vi "RT Driver VI.vi"(6 "Device Clock":string, 9 "Device Inputs FIFO":refnum<k33>, 10 "Device Outputs FIFO":refnum<k33>, 11 "Device Reference":T1 format="%.0x") -> ()   [LabVIEW 2016, in "UDP Sender Engine.lvlib"]
uses:
  UDP Sender Engine.lvlib
  <vilib>/NI Veristand/Custom Device API/Custom Device Item Ref.ctl
  <vilib>/NI Veristand/Custom Device API/Custom Device Channel Type.ctl
  Shared/Constants.vi
  <vilib>/NI Veristand/Custom Device API/Get Item Property (String).vi
  <vilib>/NI Veristand/Custom Device API/Get Item Property (U16).vi
  <vilib>/NI Veristand/Custom Device API/Custom Device API.lvlib
  <vilib>/NI Veristand/Custom Device Tools/Custom Device Utility Library/Custom Device Utility Library.lvlib
  Shared/UDP Sender Shared.lvlib
panel:
  in  "Initialization Status Notifier":refnum<notifier>
  in  "Status Notifier":refnum<notifier>
  # "Custom Device Template\nv1.0"
  # "Use this template as a starting point for creating a custom device code module. The input controls shown here are specially named controls that the system will use to provide the device loop with data. The controls are not required for the device loop to run. For instance, if the device doesn't produce any output data, then you don't need the Device Outputs FIFO control. If you do use these controls, however, they need to have these exact names to be functional."
  # "The optional status notifier element is used to notify the RT engine of the last state of the custom device, and to indicate the device has completed execution. If this control is not used, a default No Error value is returned to the system when the device finishes execution.\n\nNote: This error state is not checked until the system shuts down. Use an output status channel to send more immediate status values to the system."
  # "This optional input can be used to send the VeriStand Engine the final status of the custom device initalization process. If this control exists on the custom device front panel, the VeriStand Engine will wait for a status update before starting up. If the custom device reports an error, that will abort the execution of the current configuration in the VeriStand Engine.\n\nThis control can be deleted if the custom device does not need to send the initialization status update."
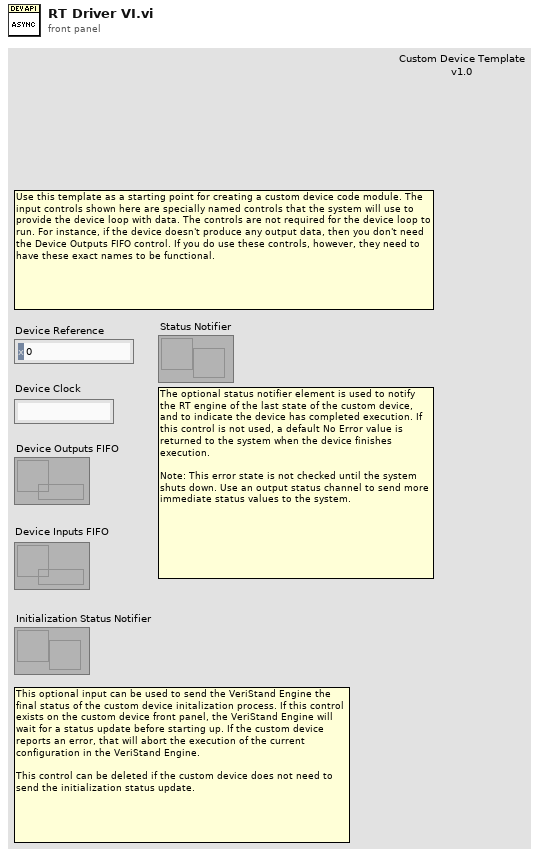
[diagram p1: front panel]
types:
  T1 = typedef "Custom Device API.lvlib/Custom Device Item Ref.ctl" = u64
  T2 = typedef "Custom Device API.lvlib/Custom Device Channel Type.ctl" = enum16{"Input", "Output"}
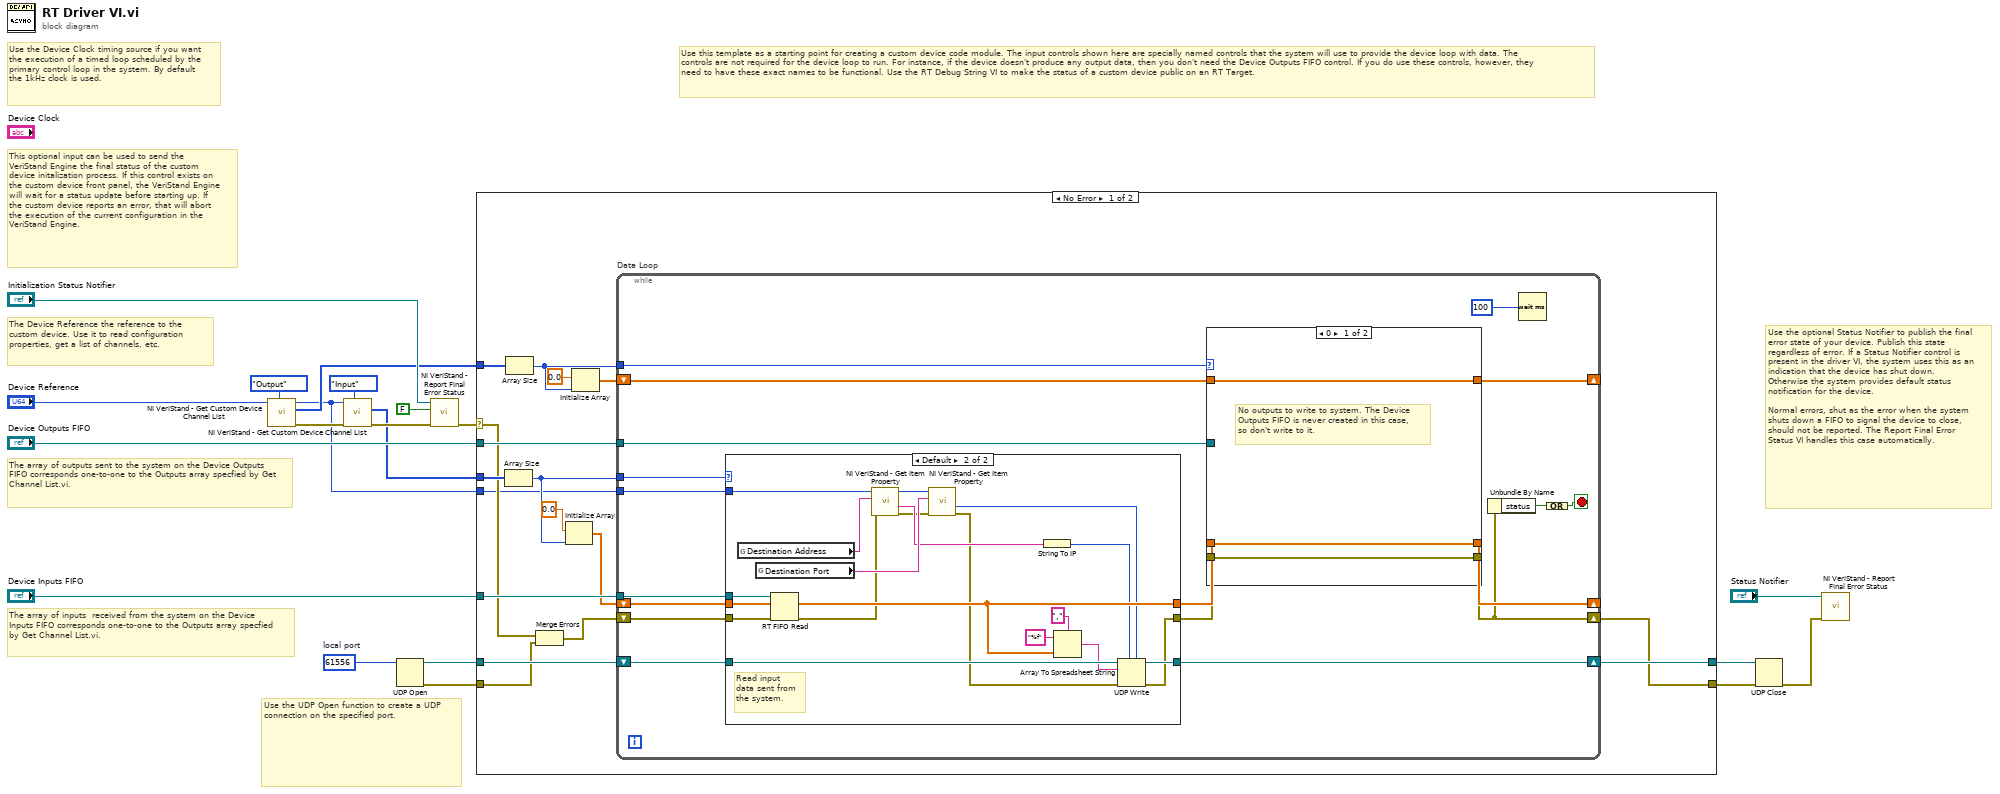
[diagram p0: block diagram]
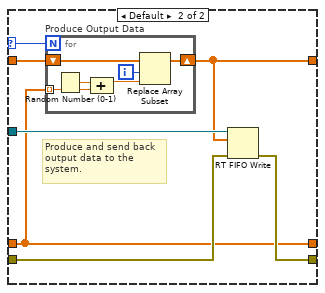
[diagram p2: hidden frame]
diagram:
  w7 = u16 61556  # local port
  # "Use the UDP Open function to create a UDP connection on the specified port."
  # "This optional input can be used to send the VeriStand Engine the final status of the custom device initalization process. If this control exists on the custom device front panel, the VeriStand Engine will wait for a status update before starting up. If the custom device reports an error, that will abort the execution of the current configuration in the VeriStand Engine."
  # "The array of inputs  received from the system on the Device Inputs FIFO corresponds one-to-one to the Outputs array specfied by Get Channel List.vi."
  # "Use the optional Status Notifier to publish the final error state of your device. Publish this state regardless of error. If a Status Notifier control is present in the driver VI, the system uses this as an indication that the device has shut down. Otherwise the system provides default status notification for the device.\n\nNormal errors, shut as the error when the system shuts down a FIFO to signal the device to close, should not be reported. The Report Final Error Status VI handles this case automatically."
  # "The array of outputs sent to the system on the Device Outputs FIFO corresponds one-to-one to the Outputs array specfied by Get Channel List.vi."
  # "The Device Reference the reference to the custom device. Use it to read configuration properties, get a list of channels, etc."
  # "Use the Device Clock timing source if you want the execution of a timed loop scheduled by the primary control loop in the system. By default the 1kHz clock is used."
  # "Use this template as a starting point for creating a custom device code module. The input controls shown here are specially named controls that the system will use to provide the device loop with data. The controls are not required for the device loop to run. For instance, if the device doesn't produce any output data, then you don't need the Device Outputs FIFO control. If you do use these controls, however, they need to have these exact names to be functional. Use the RT Debug String VI to make the status of a custom device public on an RT Target."
  n1 = call <vilib>:"NI VeriStand - Get Custom Device Channel List.vi"("Channel Type"=Custom_Device_Channel_Type."Output", "Device Ref in"="Device Reference") -> ("error out"=w15:errorcluster, "Specified Channel Ref List"=w12:T1[], "Device Ref out"=w1:T1)  [unwired: 1 in, 6 out]
  n2 = call <vilib>:"NI VeriStand - Get Custom Device Channel List.vi"("Channel Type"=Custom_Device_Channel_Type."Input", "error in (no error)"=w15, "Device Ref in"=w1) -> ("error out"=w20:errorcluster, "Specified Channel Ref List"=w13:T1[])  [unwired: 7 out]
  n3 = UDP Open(11:w7) -> (port=w6:refnum<k16>, 0:w5:errorcluster)  [unwired: 4 in, 1 out]
  n4 = call <vilib>:"NI VeriStand - Report Final Error Status.vi"("error in (no error)"=w20, "Filter FIFO & Shutdown Errors (T)"=FALSE ("Filter FIFO Errors (T)"), "Status Notifier"="Initialization Status Notifier") -> ("error out"=w9:errorcluster)  [unwired: 8 out]
  n5 = case shown="No Error" w9 {
    selector: w9 -> [w26 w96]
    tunnel: "Device Outputs FIFO" -> [w37 _]
    tunnel: "Device Inputs FIFO" -> [w36 _]
    tunnel: w13 -> [w30 _]
    tunnel: w12 -> [w29 _]
    tunnel: w6 -> [w27 w95]
    tunnel: w5 -> [w25 _]
    tunnel: [w23 w95] -> w4
    tunnel: [w22 w96] -> w3
    tunnel: w1 -> [w21 _]
    frame No Error {
      n6 = Array Size(array=w30) -> (size(s)=w28:i32)
      n7 = Array Size(array=w29) -> (size(s)=w31:i32)
      n8 = Merge Errors(w26, w25) -> (w24:errorcluster)
      n9 = Initialize Array(0.0 ("element"), w28) -> (w32:dbl[])
      n10 = Initialize Array(0.0 ("element"), w31) -> (w33:dbl[])
      n11 = while "Data Loop" {
        shift-right: [w44] -> _
        shift-left: w32 -> [w54]
        shift-right: [w39] -> w22
        shift-left: w24 -> [w55]
        shift-right: [w52] -> _
        shift-left: w33 -> [w53]
        tunnel: w31 -> [w49]
        tunnel: w37 -> [w51]
        tunnel: w36 -> [w50]
        tunnel: w28 -> [w48]
        shift-right: [w42] -> w23
        shift-left: w27 -> [w43]
        tunnel: w21 -> [w38]
        stop <- w40 stop-if-true
        n12 = case shown="Default" w48 {
          tunnel: w50 -> [_ w94]
          tunnel: w54 -> [w74 w93]
          tunnel: [w74 w86] -> w47
          tunnel: [w73 w89] -> w46
          tunnel: w55 -> [w73 w92]
          tunnel: w43 -> [w72 w91]
          tunnel: [w72 w90] -> w42
          tunnel: w38 -> [_ w81]
          frame 0 {
            # "No inputs to read\nfrom system. Inputs FIFO not created in this case, so don't write to it."
          }
          frame Default {
            # "Read input data sent from the system."
            n13 = global read "Constants.vi" "Destination Address"() -> (w83:string)
            n14 = global read "Constants.vi" "Destination Port"() -> (w82:string)
            n15 = RT FIFO Read(0:w94, 1:w93, 3:w92) -> (9:w86:dbl[], 11:w77:errorcluster)  [unwired: 4 out]
            n16 = call-poly <vilib>:"NI VeriStand - Get Item Property.vi"("error in (no error)"=w77, "Property Name"=w83, "Item Ref in"=w81) -> ("error out"=w76:errorcluster, "Value"=w78:string, "Item Ref out"=w80:T1)  [unwired: 5 in, 1 out]
            n17 = call-poly <vilib>:"NI VeriStand - Get Item Property.vi"("error in (no error)"=w76, "Property Name"=w82, "Item Ref in"=w80) -> ("error out"=w75:errorcluster, "Value"=w79:u16)  [unwired: 5 in, 2 out]
            n18 = String To IP(1:w78) -> (0:w84:u32)
            n19 = Array To Spreadsheet String(delimiter (Tab)=",", array=w86, 3:"%f" ("format string")) -> (spreadsheet string=w85:string)
            n20 = UDP Write(address=w84, port or service name=w79, connection ID=w91, data in=w85, 8:w75) -> (error out=w89:errorcluster, 3:w90:refnum<k16>)  [unwired: 1 in]
          }
        }
        n21 = case shown="0" w49 {
          selector: w49 -> [_ w59]
          tunnel: w51 -> [_ w65]
          tunnel: w53 -> [w58 w64]
          tunnel: w47 -> [w57 w60]
          tunnel: w46 -> [w56 w63]
          tunnel: [w56 w62] -> w39
          tunnel: [w58 w61] -> w52
          tunnel: [w57 w60] -> w44
          frame 0 {
            # "No outputs to write to system. The Device Outputs FIFO is never created in this case, so don't write to it."
          }
          frame Default {
            # "Produce and send back output data to the system."
            n22 = for "Produce Output Data" {
              N: w59 -> [_]
              shift-right: [w70] -> w61
              shift-left: w64 -> [w71]
              tunnel: w60 -> [w66] mode=indexing
              i -> [w69]
              n23 = Random Number (0-1)() -> (number: 0 to 1=w68:dbl)
              n24 = Compound Arithmetic op=ADD(w68, w66) -> (w67:dbl)
              n25 = Replace Array Subset(array=w71, new element=w67, index=w69) -> (w70:dbl[])
            }
            n26 = RT FIFO Write(0:w65, 1:w61, 3:w63) -> (11:w62:errorcluster)  [unwired: 1 in, 4 out]
          }
        }
        n27 = Unbundle By Name(w39) -> ("status"=w41:bool)
        n28 = Wait (ms)(milliseconds to wait=u32 100) -> ()  [unwired: 1 out]
        n29 = Compound Arithmetic op=OR(w41) -> (w40:bool)
      }
    }
    frame Error {
    }
  }
  n30 = UDP Close(connection ID=w4, 8:w3) -> (error out=w2:errorcluster)  [unwired: 1 out]
  n31 = call <vilib>:"NI VeriStand - Report Final Error Status.vi"("error in (no error)"=w2, "Status Notifier"="Status Notifier") -> ()  [unwired: 1 in, 9 out]
